vi "SetUp.vi"(8 "error in (no error)":errorcluster, 11 "Prueba06 in":refnum<class "Prueba06.lvclass">) -> (0 "error out":errorcluster, 3 "Prueba06 out":refnum<class "Prueba06.lvclass">)   [LabVIEW 2019, in "Prueba06.lvclass"]
uses:
  Prueba06.lvclass
  Prueba06.lvclass/Prueba06.ctl
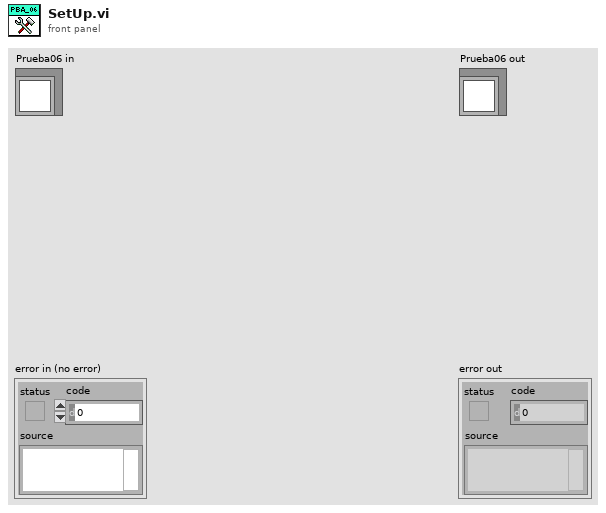
[diagram p1: front panel]
types:
  T1 = typedef "Prueba06.lvclass/BD.ctl" = cluster{"niv_presion_son_ref":dbl, "Incertidumbre":string, "Tol +":string, "Tol -":string, "max_niv_ref":dbl, "min_niv_ref":dbl}
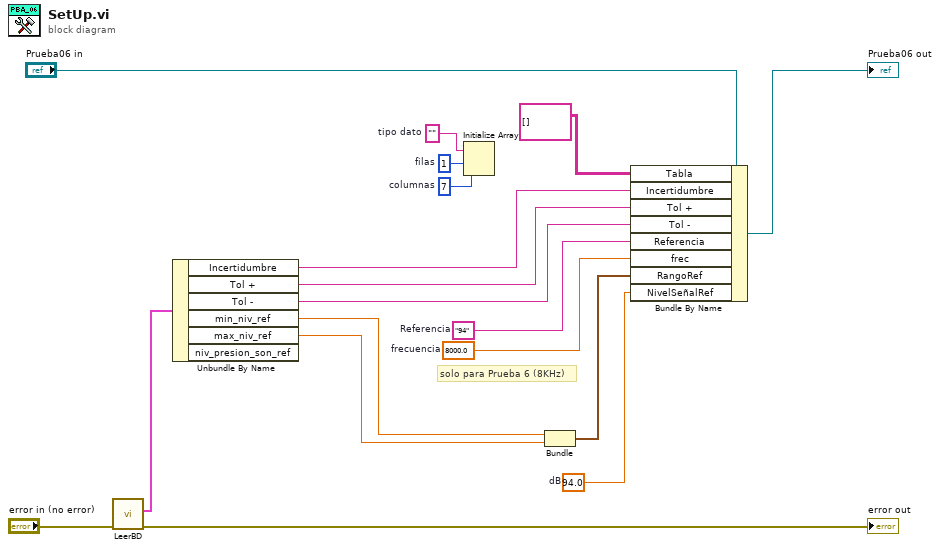
[diagram p0: block diagram]
diagram:
  w1 = 94.0  # dB
  w13 = 8000.0  # frecuencia
  w14 = "94"  # Referencia
  w16 = 7  # columnas
  w17 = 1  # filas
  w15 = ""  # tipo dato
  # "solo para Prueba 6 (8KHz)"
  n1 = call "LeerBD.vi"("error in (no error)"="error in (no error)") -> ("error out"=→"error out":errorcluster, "BD"=w7:T1)  [unwired: 8 in, 1 out]
  n2 = Unbundle By Name(w7) -> ("Incertidumbre"=w6:string, "Tol +"=w5:string, "Tol -"=w4:string, "min_niv_ref"=w3:dbl, "max_niv_ref"=w2:dbl)  [unwired: 1 out]
  n3 = Initialize Array(w15, w17, w16) -> ()  [unwired: 1 out]
  n4 = Bundle("min_niv_ref"=w3, "max_niv_ref"=w2) -> (w10:cluster{"min_niv_ref":dbl, "max_niv_ref":dbl})  [unwired: 1 in]
  n5 = Bundle By Name(cluster="Prueba06 in", "Tabla"=string[][] [], "Incertidumbre"=w6, "Tol +"=w5, "Tol -"=w4, "Referencia"=w14, "frec"=w13, "RangoRef"=w10, "NivelSeñalRef"=w1) -> (→"Prueba06 out":refnum<class "Prueba06.lvclass">)
